vi "Write nextInChain.vi"(8 "error in (no error)":errorcluster, 10 "Chain.lvclass":refnum<class "Chain.lvclass">, 11 "Subtract in":refnum<class "Subtract.lvclass">) -> (0 "error out":errorcluster, 3 "Subtract out":refnum<class "Subtract.lvclass">)   [LabVIEW 2017, in "Subtract.lvclass"]
uses:
  Subtract.lvclass
  Chain Class/Chain.lvclass
  Subtract.lvclass/Subtract.ctl
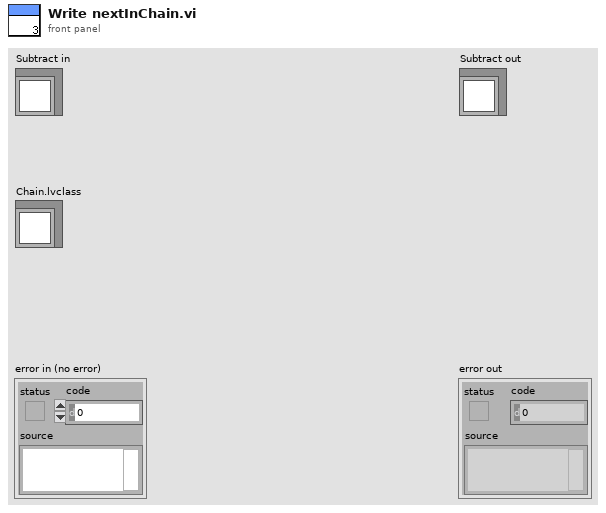
[diagram p1: front panel]
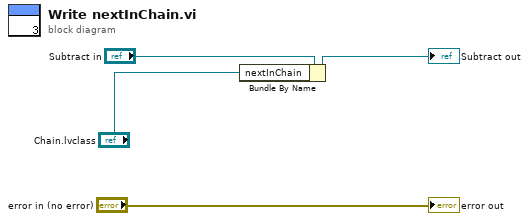
[diagram p0: block diagram]
diagram:
  n1 = Bundle By Name(cluster="Subtract in", "nextInChain"="Chain.lvclass") -> (→"Subtract out":refnum<class "Subtract.lvclass">)
  "error out" <- "error in (no error)"
